vi "试剂余量后台任务.vi"   [LabVIEW 2016, in "斯坦道CODMn新电路板.lvlib"]
types:
  T1 = cluster{"V1":sgl, "V2":sgl, "V3":sgl, "V4":sgl, "V5":sgl, "V6":sgl, "V7":sgl, "V8":sgl, "V9":sgl, "V10":sgl, "V11":sgl, "V12":sgl, "V9-1":sgl, "V9-2":sgl}
  T2 = typedef "量程选择控件.ctl" = enum32{"L", "H", "AUTO"}
  T3 = cluster{"水样测试量程模式":T2, "标样核查量程模式":T2, "零点核查量程模式":T2, "跨度核查量程模式":T2, "空白测试量程模式":T2, "平行样测试量程模式":T2, "加标回收量程模式":T2, "空白校准量程模式":T2, "标样校准量程模式":T2}
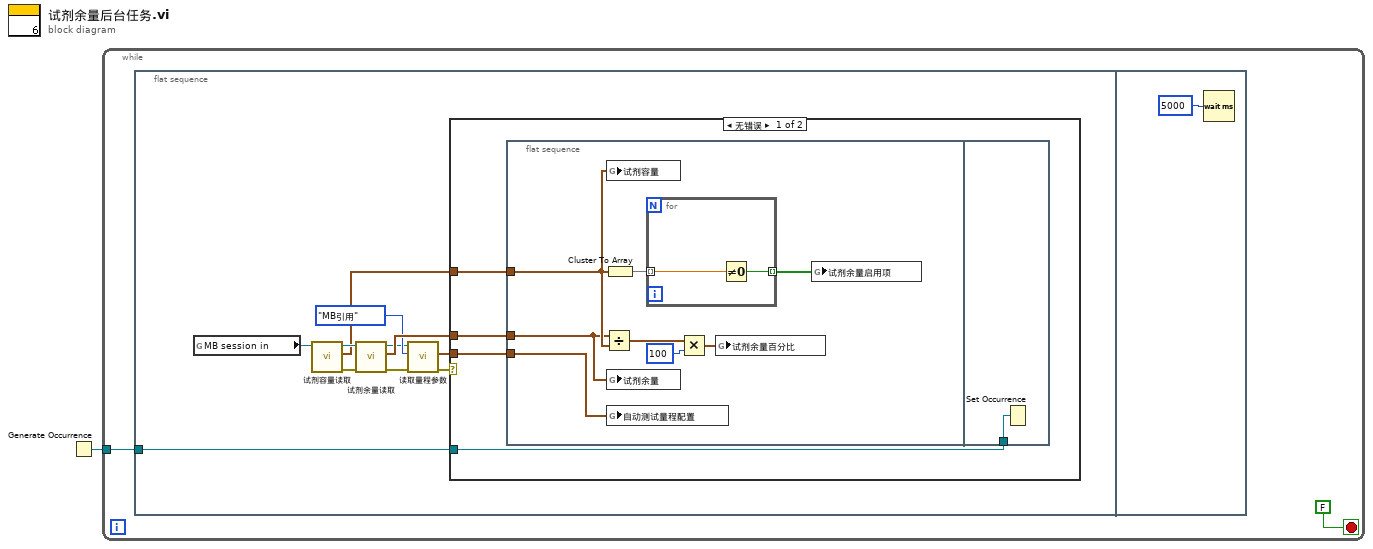
[diagram p0: block diagram]
diagram:
  n1 = Generate Occurrence() -> (w1:refnum<k4>)
  n2 = while {
    tunnel: w1 -> [w2]
    stop <- FALSE stop-if-true
    n3 = flat-sequence {
      tunnel: w2 -> [w9]
      frame #0 {
        n4 = global read "VARCODMn全局变量.vi" "MB session in"() -> (w12:refnum<class "MB_Master.lvclass">)
        n5 = call "试剂容量读取.vi"("MB session in"=w12) -> ("error out"=w14:errorcluster, "试剂容量"=w11:T1, "MB session out"=w13:refnum<class "MB_Master.lvclass">)  [unwired: 8 in]
        n6 = call "试剂余量读取.vi"("Error in"=w14, "MB session in"=w13) -> ("error out"=w5:errorcluster, "试剂余量"=w10:T1, "MB session out"=w7:refnum<class "MB_Master.lvclass">)  [unwired: 7 in]
        n7 = call "读取量程参数.vi"("error in (no error)"=w5, "引用选择"=enum16{"MB引用", "自建引用"}."MB引用", "MB session in"=w7) -> ("error out"=w4:errorcluster, "自动测试量程配置"=w6:T3)  [unwired: 6 in, 1 out]
        n8 = case shown="无错误" w4 {
          tunnel: w11 -> [w18 _]
          tunnel: w10 -> [w17 _]
          tunnel: w9 -> [w16 _]
          tunnel: w6 -> [w15 _]
          frame No Error {
            n9 = flat-sequence {
              tunnel: w18 -> [w24]
              tunnel: w17 -> [w23]
              tunnel: w15 -> [w19]
              tunnel: w16 -> [w29]
              frame #0 {
                n10 = Divide(x=w23, y=w24) -> (x/y=w26:T1)
                n11 = Cluster To Array(cluster=w24) -> (array=w21:sgl[])
                n12 = global write "VARCODMn全局变量.vi" "试剂容量"(w24) -> ()
                n13 = global write "VARCODMn全局变量.vi" "试剂余量"(w23) -> ()
                n14 = global write "CODMn断电保存全局变量.vi" "自动测试量程配置"(w19) -> ()
                n15 = for {
                  tunnel: w21 -> [w28] mode=indexing
                  tunnel: [w27] -> w20 mode=indexing
                  n16 = Not Equal To 0?(x=w28) -> (x != 0?=w27:bool)
                }
                n17 = Multiply(x=w26, y=100) -> (x*y=w22:T1)
                n18 = global write "VARCODMn全局变量.vi" "试剂余量百分比"(w22) -> ()
                n19 = global write "VARCODMn全局变量.vi" "试剂余量启用项"(w20) -> ()
              }
              frame #1 {
                n20 = Set Occurrence(w29) -> ()
              }
            }
          }
          frame Error {
          }
        }
      }
      frame #1 {
        n21 = Wait (ms)(milliseconds to wait=u32 5000 ("等待时间（毫秒）")) -> ()  [unwired: 1 out]
      }
    }
  }
